vi "diagramdisable.vi"() -> ()   [LabVIEW 2013]
panel:
  in  "stop":bool
  out "product":dbl(knob) scale=0.0..200.0
  out "sum":dbl(knob) scale=0.0..50.0
  in  "a":dbl(slide) scale=0.0..10.0
  in  "b":dbl(slide) scale=0.0..10.0
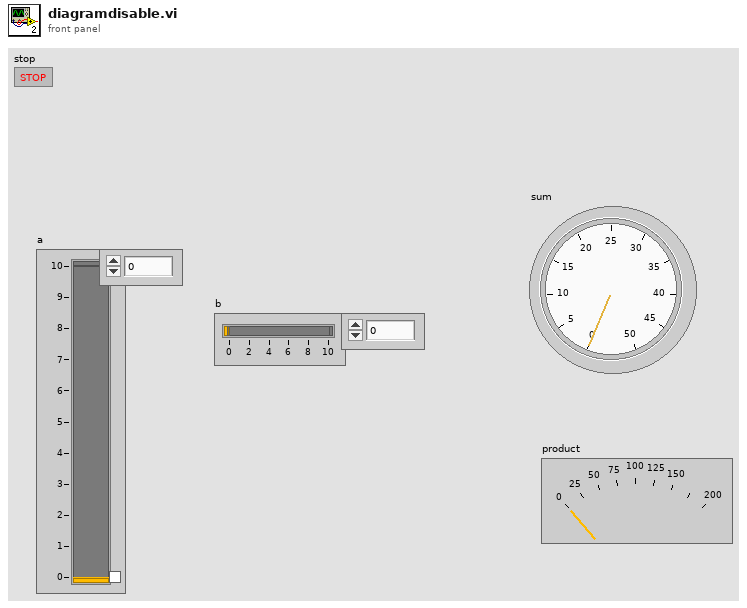
[diagram p1: front panel]
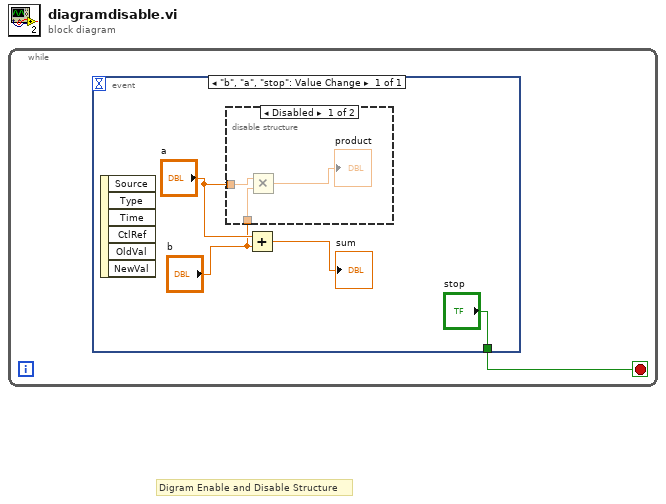
[diagram p0: block diagram]
diagram:
  # "Digram Enable and Disable Structure"
  n1 = while {
    stop <- w1 stop-if-true
    n2 = event shown="[0] \"b\", \"a\", \"stop\": Value Change" {
      selector: _ -> [_]
      dyn-events: _ -> [_]
      timeout: _ -> [_]
      tunnel: ["stop"] -> w1
      event "b", "a", "stop": Value Change {
        n3 = event-data() -> ()  [unwired: 1 in, 6 out]
        n4 = disable-structure shown="Disabled" {
          disable-tunnel: "a" -> [w8 _]
          disable-tunnel: "b" -> [w7 _]
          frame Disabled {
            n5 = Multiply(x=w8, y=w7) -> (x*y=→"product":dbl)
          }
          frame Enabled {
          }
        }
        n6 = Add(x="a", y="b") -> (x+y=→"sum":dbl)
      }
    }
  }
